vi "Find Xbee State Machine.vi"(11 "Incoming Bytes":u8) -> (3 "Xbee Found":bool)   [LabVIEW 2014]
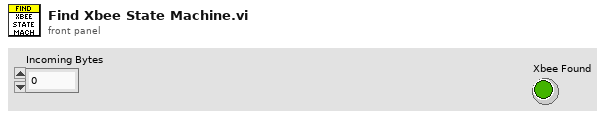
[diagram p1: front panel]
types:
  T1 = enum16{"Waiting For Start Byte", "Calculate Message Size", "Build Message"}
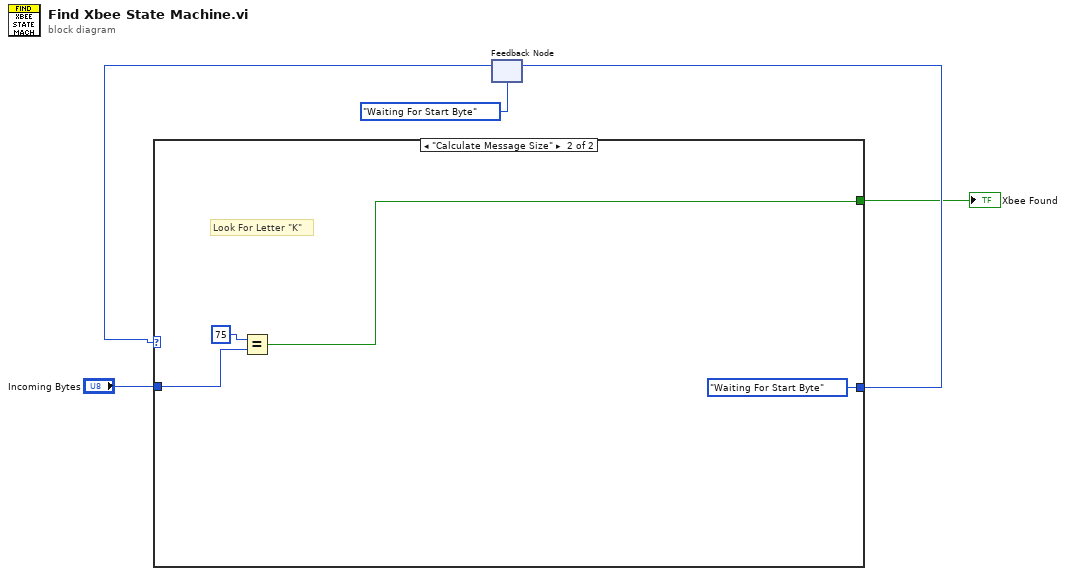
[diagram p0: block diagram]
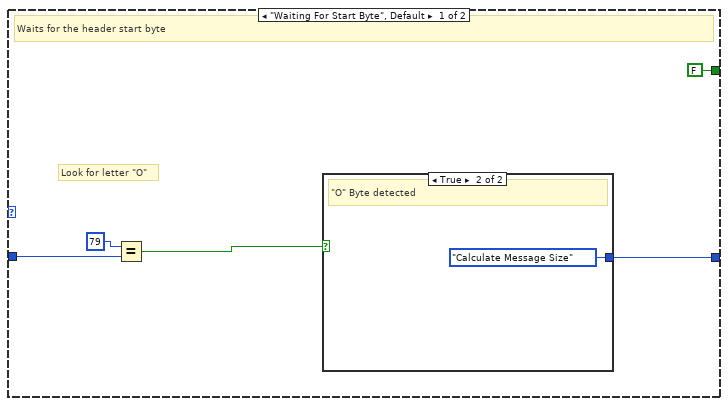
[diagram p2: hidden frame]
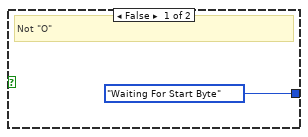
[diagram p3: hidden frame]
diagram:
  n1 = feedback #1(T1."Waiting For Start Byte" ("Message States")) -> (w4:T1)
  n2 = case shown="\"Calculate Message Size\"" w4 {
    tunnel: "Incoming Bytes" -> [w8 w14]
    tunnel: [w7 T1."Waiting For Start Byte" ("Message States")] -> w2
    tunnel: [FALSE w13] -> w1
    frame "Waiting For Start Byte", Default {
      # "Look for letter \"O\""
      # "Waits for the header start byte"
      n3 = Equal?(x=u8 79, y=w8) -> (x = y?=w9:bool)
      n4 = case shown="True" w9 {
        tunnel: [T1."Waiting For Start Byte" ("Message States") T1."Calculate Message Size" ("Message States")] -> w7
        frame False {
          # "Not \"O\""
        }
        frame True {
          # "\"O\" Byte detected"
        }
      }
    }
    frame "Calculate Message Size" {
      # "Look For Letter \"K\""
      n5 = Equal?(x=u8 75, y=w14) -> (x = y?=w13:bool)
    }
  }
  "Xbee Found" <- w1
  n6 = feedback-in #1(w2) -> ()
